vi "SpliParameter.vi"(1 "Parameter":string) -> (0 "Output":string[](array[string]))   [LabVIEW 2010]
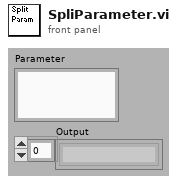
[diagram p1: front panel]
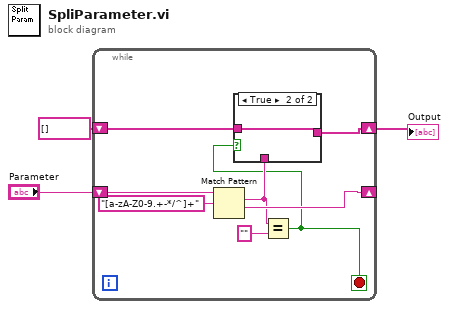
[diagram p0: block diagram]
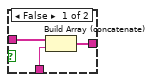
[diagram p2: hidden frame]
diagram:
  n1 = while {
    shift-right: [w9] -> _
    shift-left: "Parameter" -> [w11]
    shift-right: [w5] -> w1
    shift-left: string[] [] -> [w7]
    stop <- w4 stop-if-true
    n2 = Match Pattern(string=w11, regular expression="[a-zA-Z0-9.+-*/^]+") -> (match substring=w6:string, after substring=w9:string)  [unwired: 1 in, 2 out]
    n3 = Equal?(x=w6, y="") -> (x = y?=w4:bool)
    n4 = case shown="True" w4 {
      tunnel: w7 -> [w14 w15]
      tunnel: w6 -> [w13 _]
      tunnel: [w12 w15] -> w5
      frame False {
        n5 = Build Array (concatenate)(w14, w13) -> (w12:string[])
      }
      frame True {
      }
    }
  }
  "Output" <- w1
